vi "Média últimos 4 números - shift register com multiplas entradas.vi"() -> ()   [LabVIEW 2018]
panel:
  out "Waveform Chart":dynamicdata(graph)
  out "Média últimos 4 números":dbl
  out "Dados actuais":dbl
  out "Nº Ciclo":i32
  in  "stop":bool
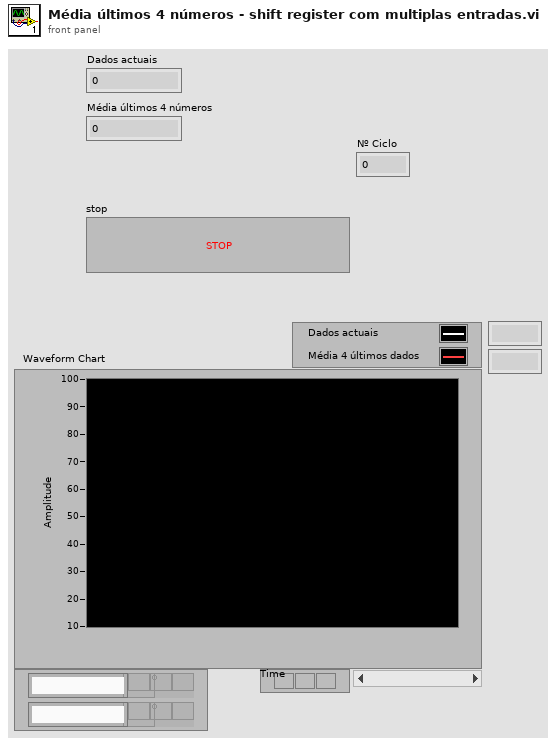
[diagram p1: front panel]
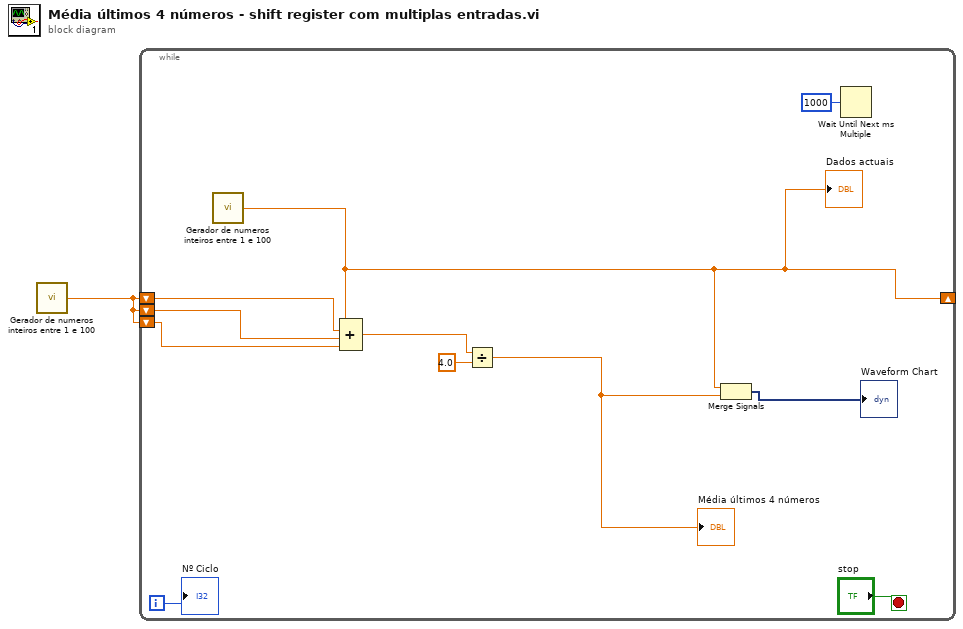
[diagram p0: block diagram]
diagram:
  n1 = call "Gerador de numeros inteiros entre 1 e 100.vi"() -> ("Numeric"=w1:dbl)
  n2 = while {
    shift-right: [w3] -> _
    shift-left: w1 -> [w9]
    shift-left: w1 -> [w8]
    shift-left: w1 -> [w7]
    i -> [w10]
    stop <- "stop" stop-if-true
    n3 = call "Gerador de numeros inteiros entre 1 e 100.vi"() -> ("Numeric"=w3:dbl)
    "Dados actuais" <- w3
    n4 = Compound Arithmetic op=ADD(w3, w9, w8, w7) -> (w6:dbl)
    n5 = Divide(x=w6, y=4.0) -> (x/y=w4:dbl)
    "Média últimos 4 números" <- w4
    n6 = Merge Signals(w3, w4) -> (→"Waveform Chart":dynamicdata)
    n7 = Wait Until Next ms Multiple(millisecond multiple=u32 1000) -> ()  [unwired: 1 out]
    "Nº Ciclo" <- w10
  }
